vi "Modules Processes.vi"(8 "error in (no error)":errorcluster) -> (0 "error out":errorcluster)   [LabVIEW 2020]
uses:
  Test Driver/Test Driver.lvlib
  Motion/Motion.lvlib
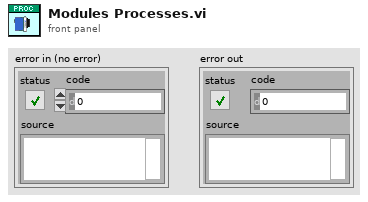
[diagram p1: front panel]
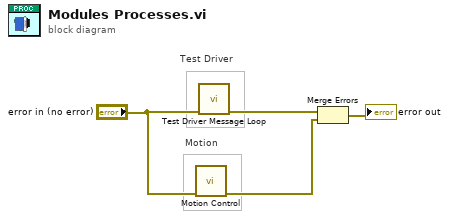
[diagram p0: block diagram]
diagram:
  # "Motion"
  # "Test Driver"
  n1 = call "Motion Control.vi"("error in (no error)"="error in (no error)") -> ("error out"=w2:errorcluster)  [unwired: 10 in]
  n2 = call "Test Driver Message Loop.vi"("error in (no error)"="error in (no error)") -> ("error out"=w3:errorcluster)  [unwired: 10 in]
  n3 = Merge Errors(w3, w2) -> (→"error out":errorcluster)
